vi "task_3.vi"() -> ()   [LabVIEW 2020]
panel:
  out "Top 3":cluster{"Player1":string, "Score":i32}[](array[cluster])
  out "Player Info":cluster{"Player1":string, "Score":i32}
  in  "Blue":bool
  out "Blue LED":bool
  in  "Red":bool
  out "Red LED":bool
  in  "Green":bool
  out "Green LED":bool
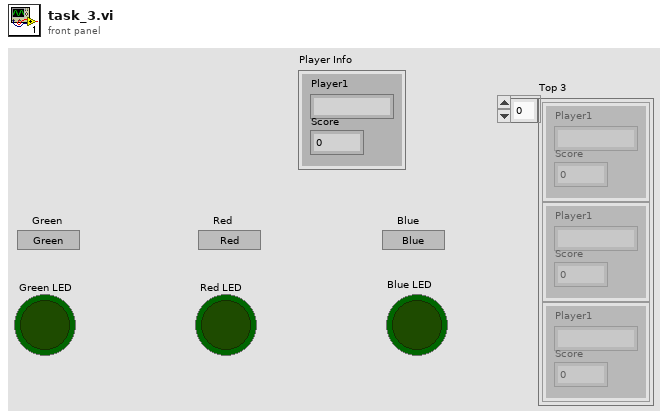
[diagram p1: front panel]
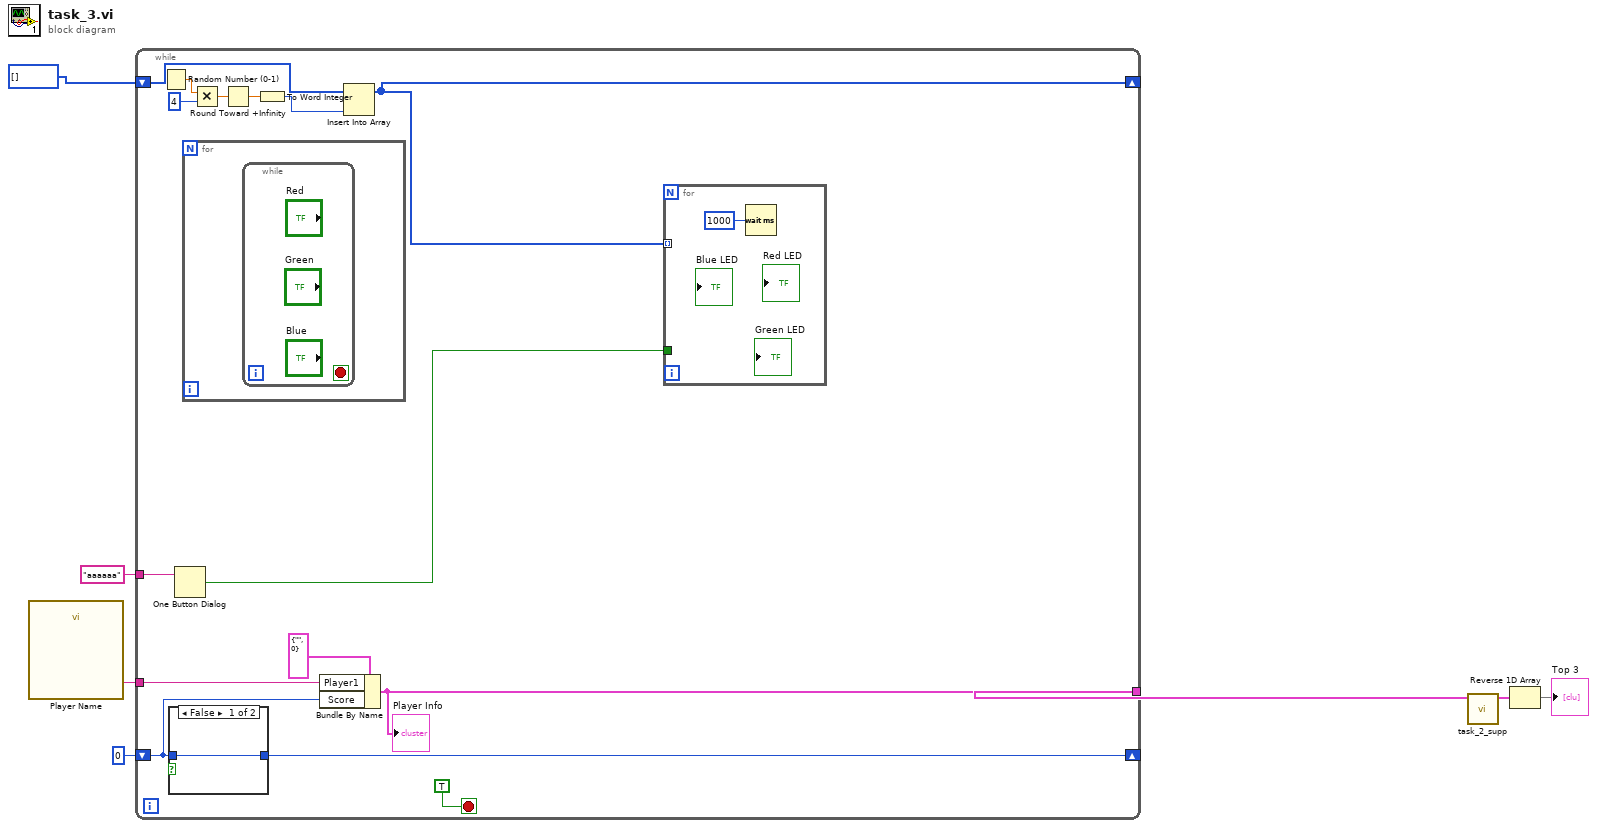
[diagram p0: block diagram]
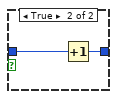
[diagram p2: hidden frame]
diagram:
  n1 = call "Player Name"() -> ("name"=w4:string)  [unwired: 17 in, 2 out]
  n2 = while {
    tunnel: [w16] -> w5
    tunnel: w4 -> [w15]
    shift-right: [w13] -> _
    shift-left: 0 -> [w14]
    tunnel: "aaaaaa" -> [w12]
    shift-right: [w8] -> _
    shift-left: i32[] [] -> [w9]
    stop <- TRUE stop-if-true
    n3 = Random Number (0-1)() -> (number: 0 to 1=w22:dbl)
    n4 = case shown="False" {
      selector: _ -> [_ _]
      tunnel: w14 -> [w23 w25]
      tunnel: [w23 w24] -> w13
      frame False {
      }
      frame True {
        n5 = Increment(x=w25) -> (x+1=w24:i32)
      }
    }
    n6 = One Button Dialog(message=w12) -> (true=w11:bool)  [unwired: 1 in]
    n7 = for {
      n8 = while {
        stop <- _ stop-if-true
      }
    }
    n9 = Multiply(x=w22, y=4) -> (x*y=w21:dbl)
    n10 = Round Toward +Infinity(x=w21) -> (ceil(x): smallest int >= x=w19:dbl)
    n11 = To Word Integer(number=w19) -> (16bit integer=w10:i16)
    n12 = Bundle By Name(cluster=cluster{"Player1":string, "Score":i32} {"Player1"="", "Score"=0} ("Player Info"), "Player1"=w15, "Score"=w14) -> (w16:cluster{"Player1":string, "Score":i32})
    "Player Info" <- w16
    n13 = Insert Into Array(array=w9, new element=w10) -> (w8:i32[])  [unwired: 1 in]
    n14 = for {
      tunnel: w11 -> [_]
      tunnel: w8 -> [_] mode=indexing
      n15 = Wait (ms)(milliseconds to wait=1000) -> ()  [unwired: 1 out]
    }
  }
  n16 = call "task_2_supp.vi"("Player Info"=w5) -> ("Array"=w7:cluster{"Player1":string, "Score":i32}[])  [unwired: 10 in]
  n17 = Reverse 1D Array(array=w7) -> (reversed array=→"Top 3":cluster{"Player1":string, "Score":i32}[])
